vi "LogArray.vi"(6 "Values":i32[](array[numeric])=[1, 2, 3], 7 "Alarm?":bool=TRUE, 8 "Name":string="Acceleration: ") -> (2 "Log String":string, 5 "Log Array":string[](array[string]))   [LabVIEW 2013]
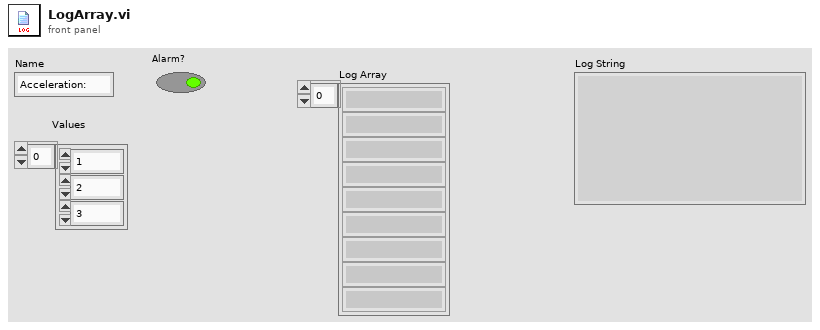
[diagram p1: front panel]
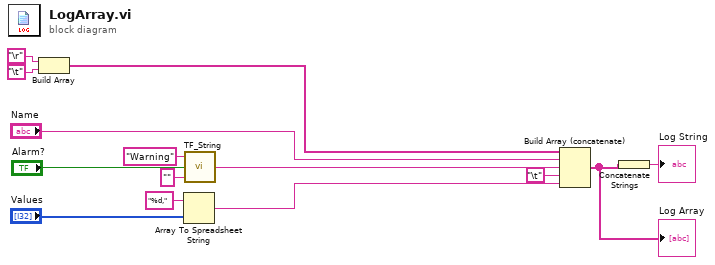
[diagram p0: block diagram]
diagram:
  n1 = Build Array("\r", "\t") -> (w8:string[])
  n2 = Array To Spreadsheet String(array="Values", 3:"%d," ("format string")) -> (spreadsheet string=w5:string)  [unwired: 1 in]
  n3 = call "TF_String.vi"("FalseCase"="", "Case"="Alarm?", "TrueCase"="Warning") -> ("Result"=w10:string)
  n4 = Build Array (concatenate)(w8, "Name", w10, "\t", w5) -> (w2:string[])
  "Log Array" <- w2
  n5 = Concatenate Strings(w2) -> (→"Log String":string)
